vi "Receive Data from ESP32.vi"() -> ()   [LabVIEW 2018]
panel:
  out "name 2":string
  out "net address":u32[](array[numeric])
  out "name":string
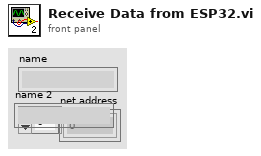
[diagram p1: front panel]
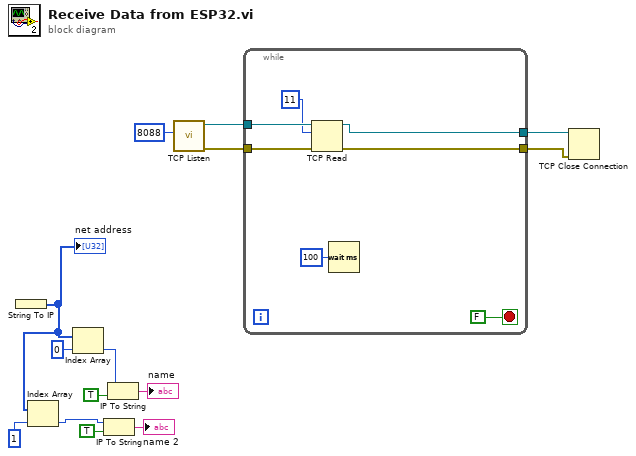
[diagram p0: block diagram]
diagram:
  n1 = String To IP() -> (0:w2:u32[])  [unwired: 1 in]
  "net address" <- w2
  n2 = Index Array(array=w2, index=1) -> (element=w1:u32)
  n3 = Index Array(array=w2, index=0) -> (element=w7:u32)
  n4 = IP To String(1:TRUE ("dot notation? (F)"), 2:w1) -> (0:→"name 2":string)
  n5 = IP To String(1:TRUE ("dot notation? (F)"), 2:w7) -> (0:→"name":string)
  n6 = call <vilib>:"TCP Listen.vi"("port"=u16 8088) -> ("error out"=w12:errorcluster, "connection ID"=w13:refnum<k5>)  [unwired: 6 in, 3 out]
  n7 = while {
    tunnel: w13 -> [w21]
    tunnel: w12 -> [w18]
    tunnel: [w17] -> w11
    tunnel: [w16] -> w10
    stop <- FALSE stop-if-true
    n8 = TCP Read(connection ID=w21, bytes to read=11, error in (no error)=w18) -> (connection ID out=w17:refnum<k5>, error out=w16:errorcluster)  [unwired: 3 out]
    n9 = Wait (ms)(milliseconds to wait=u32 100) -> ()  [unwired: 1 out]
  }
  n10 = TCP Close Connection(connection ID=w11, error in (no error)=w10) -> ()  [unwired: 1 in, 2 out]
